vi "Load Store Instrument Setup.vi"(8 "error in (no error)":errorcluster, 9 "File Name":string, 10 "Operation Type (0: Load)":i32(ring) items=["Load", "Store"], 11 "VISA resource name":refnum<visa-resource-name>) -> (0 "error out":errorcluster, 3 "VISA resource name out":refnum<visa-resource-name>)   [LabVIEW 2012, in "Keysight B2980 Series.lvlib"]
doc: "Loads or saves the instrument setup from or to the specified file in the current directory."
uses:
  Keysight B2980 Series.lvlib
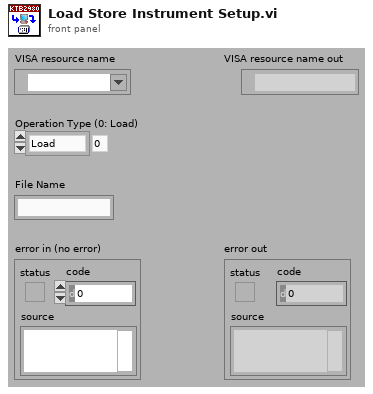
[diagram p1: front panel]
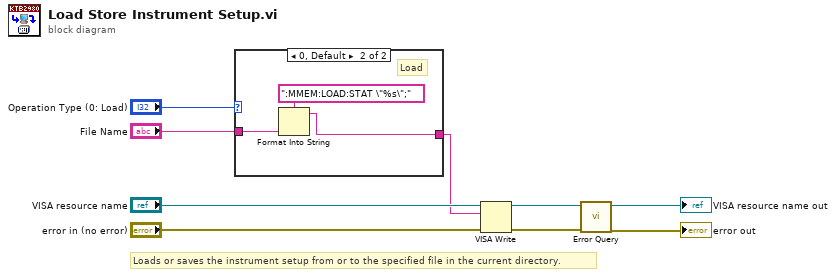
[diagram p0: block diagram]
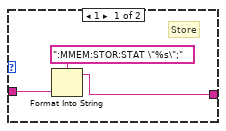
[diagram p2: hidden frame]
diagram:
  # "Loads or saves the instrument setup from or to the specified file in the current directory."
  n1 = case shown="0, Default" "Operation Type (0: Load)" {
    tunnel: "File Name" -> [w11 w14]
    tunnel: [w10 w13] -> w1
    frame 1 {
      # "Store"
      n2 = Format Into String(format string=":MMEM:STOR:STAT \"%s\";", w11) -> (resulting string=w10:string)  [unwired: 2 in, 1 out]
    }
    frame 0, Default {
      # "Load"
      n3 = Format Into String(format string=":MMEM:LOAD:STAT \"%s\";", w14) -> (resulting string=w13:string)  [unwired: 2 in, 1 out]
    }
  }
  n4 = VISA Write(VISA resource name="VISA resource name", write buffer=w1, error in (no error)="error in (no error)") -> (VISA resource name out=w6:refnum<visa-resource-name>, error out=w5:errorcluster)  [unwired: 1 out]
  n5 = call "Error Query.vi"("error in (no error)"=w5, "VISA resource name"=w6) -> ("error out"=→"error out":errorcluster, "VISA resource name out"=→"VISA resource name out":refnum<visa-resource-name>)  [unwired: 8 out]
